vi "Read SBOM Components from VIPM Project Scan.vi"(8 "error in (no error)":errorcluster, 11 "LabVIEW project path":path) -> (0 "error out":errorcluster, 3 "SBOM Components out":refnum<class "CycloneDX Component.lvclass">[](array[class]))   [LabVIEW 2017, in "VIP SBOM Support.lvlib"]
doc: "Scans a LabVIEW project for package dependencies and generate a list of CycloneDX SBOM components."
uses:
  VIP SBOM Support.lvlib
  CycloneDX/CycloneDX Component/CycloneDX Component.lvclass
  <vilib>/JKI/VIPM API/VIPM API_vipm_api.lvlib
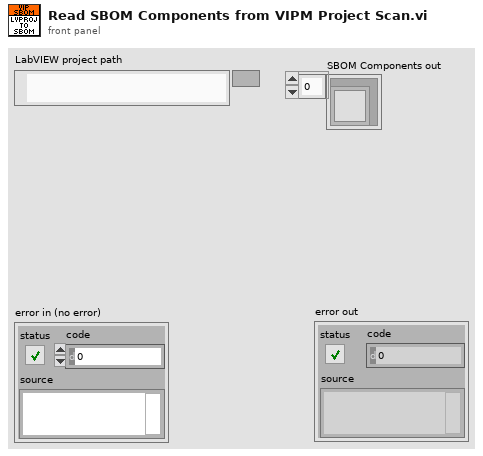
[diagram p1: front panel]
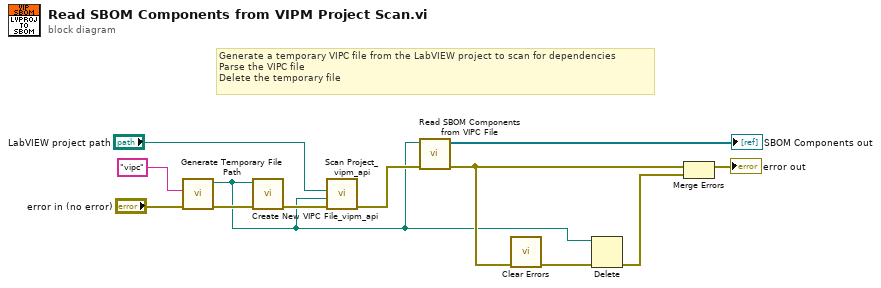
[diagram p0: block diagram]
diagram:
  # "Generate a temporary VIPC file from the LabVIEW project to scan for dependencies\nParse the VIPC file\nDelete the temporary file"
  n1 = call <vilib>:"Generate Temporary File Path.vi"("error in (no error)"="error in (no error)", "Temporary File Extension (tmp)"="vipc") -> ("error out"=w7:errorcluster, "Unique Temporary File Path"=w1:path)  [unwired: 8 in]
  n2 = call <vilib>:"Create New VIPC File_vipm_api.vi"("error in (no error)"=w7, "Path to New VIPC File"=w1) -> ("error out"=w10:errorcluster)  [unwired: 9 in]
  n3 = call <vilib>:"Scan Project_vipm_api.vi"("error in (no error)"=w10, "Path to VIPC File"=w1, "Project file, VI or project dir path"="LabVIEW project path") -> ("error out"=w12:errorcluster)  [unwired: 8 in]
  n4 = call "Read SBOM Components from VIPC File.vi"("error in (no error)"=w12, "VIPC path"=w1) -> ("error out"=w5:errorcluster, "SBOM Components out"=→"SBOM Components out":refnum<class "CycloneDX Component.lvclass">[])  [unwired: 8 in]
  n5 = call <vilib>:"Clear Errors.vi"("error in (no error)"=w5) -> ("error out"=w4:errorcluster)  [unwired: 5 in, 1 out]
  n6 = Delete(path (use dialog)=w1, error in=w4) -> (error out=w2:errorcluster)  [unwired: 3 in, 2 out]
  n7 = Merge Errors(w5, w2) -> (→"error out":errorcluster)
